vi "Analyze Waveform.vi"(8 "error in (no error)":errorcluster, 9 "Pulse Count (1)":i32=1, 10 "Target Channel":string, 11 "CapturedData":waveform(dbl)[](array[waveform])) -> (0 "error out":errorcluster, 1 "PulseAnalysis":T1[](array[typedef]), 2 "MissingPulse":bool, 3 "MissingChannel":bool)   [LabVIEW 2019, in "Variant Parser.lvlib" / "WaveformProcessor.lvclass"]
uses:
  Library/WaveformProcessor.lvclass
  Custom Controls/Pulse Analysis.ctl
  Library/WaveformProcessor.lvclass/WaveformProcessor.ctl
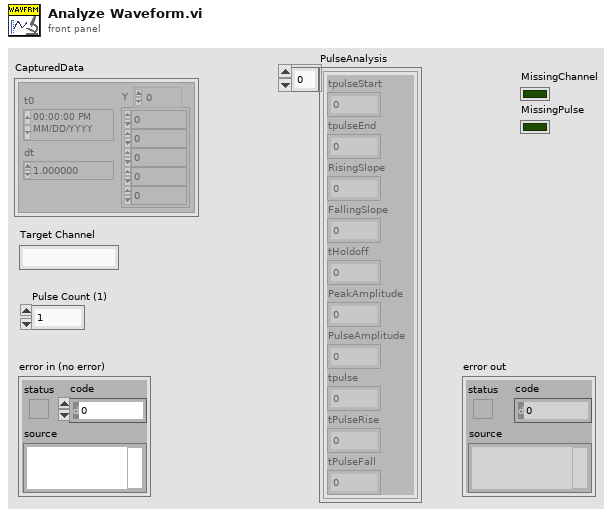
[diagram p1: front panel]
types:
  T1 = typedef "Variant Parser.lvlib/WaveformProcessor.lvclass/Pulse Analysis.ctl" = cluster{"tpulseStart":dbl, "tpulseEnd":dbl, "RisingSlope":dbl, "FallingSlope":dbl, "tHoldoff":dbl, "PeakAmplitude":dbl, "PulseAmplitude":dbl, "tpulse":dbl, "tPulseRise":dbl, "tPulseFall":dbl}
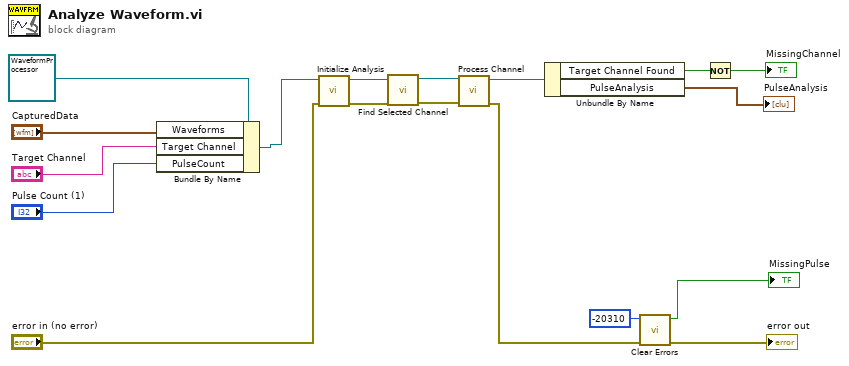
[diagram p0: block diagram]
diagram:
  n1 = Bundle By Name(cluster=refnum<class "WaveformProcessor.lvclass"> refnum ("Variant Parser.lvlib:WaveformProcessor.lvclass"), "Waveforms"="CapturedData", "Target Channel"="Target Channel", "PulseCount"="Pulse Count (1)") -> (w11:refnum<class "WaveformProcessor.lvclass">)
  n2 = call "Initialize Analysis.vi"("error in (no error)"="error in (no error)", "WaveformProcessor in"=w11) -> ("error out"=w12:errorcluster, "WaveformProcessor out"=w15:refnum<class "WaveformProcessor.lvclass">)  [unwired: 8 in]
  n3 = call "Find Selected Channel.vi"("error in (no error)"=w12, "WaveformProcessor in"=w15) -> ("error out"=w13:errorcluster, "WaveformProcessor out"=w14:refnum<class "WaveformProcessor.lvclass">)  [unwired: 8 in]
  n4 = call "Process Channel.vi"("error in"=w13, "WaveformProcessor"=w14) -> ("error out"=w4:errorcluster, "WaveformProcessor out"=w9:refnum<class "WaveformProcessor.lvclass">)  [unwired: 8 in]
  n5 = Unbundle By Name(w9) -> ("Target Channel Found"=w8:bool, "PulseAnalysis"=→"PulseAnalysis":T1[])
  n6 = call <vilib>:"Clear Errors.vi"("error in (no error)"=w4, "specific error code to clear (0: all)"=-20310) -> ("error out"=→"error out":errorcluster, "specific error cleared?"=→"MissingPulse":bool)  [unwired: 4 in]
  n7 = Not(x=w8) -> (.not. x?=→"MissingChannel":bool)
